vi "update.vi"(8 "error in (no error)":errorcluster, 10 "model":refnum<class "Model.lvclass">, 11 "AutomatedMotionState in":refnum<class "AutomatedMotionState.lvclass">) -> (0 "error out":errorcluster, 2 "model 2":refnum<class "Model.lvclass">, 3 "AutomatedMotionState out":refnum<class "AutomatedMotionState.lvclass">)   [LabVIEW 2013, in "AutomatedMotionState.lvclass"]
uses:
  AutomatedMotionState.lvclass
  Model/Model/Model.lvclass
  ControlledMotionState/ControlledMotionState.lvclass
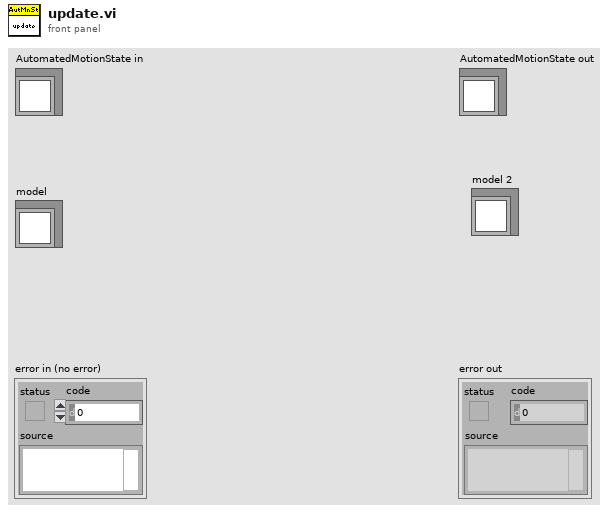
[diagram p1: front panel]
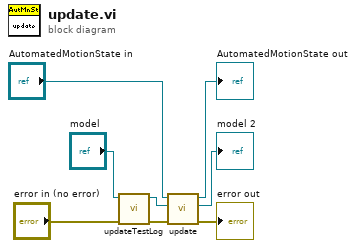
[diagram p0: block diagram]
diagram:
  n1 = call "updateTestLog.vi"("error in (no error)"="error in (no error)", "Model in"="model") -> ("error out"=w3:errorcluster, "Model out"=w1:refnum<class "Model.lvclass">)  [unwired: 8 in]
  n2 = call-parent "update.vi"("error in (no error)"=w3, "model"=w1, "ControlledMotionState in"="AutomatedMotionState in") -> ("error out"=→"error out":errorcluster, "model 2"=→"model 2":refnum<class "Model.lvclass">, "ControlledMotionState out"=→"AutomatedMotionState out":refnum<class "AutomatedMotionState.lvclass">)  [unwired: 6 in]
